vi "Report Data Update the Caller.vi"(8 "error in (no error)":errorcluster, 10 "Report Data":T1={"Schema"="", "Test Socket"="", "Start Test Cycle"="", "Stop Test Cycle"="", "Test Mode"="", "Frame Type"="fe_frame_log"}, 11 "Post Analysis in":refnum<class "Post Analysis.lvclass">) -> (0 "error out":errorcluster, 3 "Post Analysis out":refnum<class "Post Analysis.lvclass">)   [LabVIEW 2023, in "Data Analysis.lvlib" / "Post Analysis.lvlib" / "Post Analysis.lvclass"]
uses:
  Post Analysis.lvclass
  Control/Report.ctl
  Post Analysis.lvclass/Post Analysis.ctl
  Test Info/Test Info Messages/Report Data Update the Self Msg/Report Data Update the Self Msg.lvclass/Report Data Update the Self Msg.ctl
  <vilib>/ActorFramework/Message Enqueuer/Message Enqueuer.lvclass/Message Enqueuer.ctl
  Error Log/Error Log Messages/Result Data Update the Self Msg/Result Data Update the Self Msg.lvclass/Result Data Update the Self Msg.ctl
  FE FF Frame/FE FF Frame Messages/Result Data Update the Self Msg/Result Data Update the Self Msg.lvclass/Result Data Update the Self Msg.ctl
  Signal Analysis/Signal Analysis Messages/Result Data Update the Self Msg/Result Data Update the Self Msg.lvclass/Result Data Update the Self Msg.ctl
  Import Export/Import Export Messages/Result Data Update the Self Msg/Result Data Update the Self Msg.lvclass/Result Data Update the Self Msg.ctl
  Result Info/Result Info Messages/Result Data Update the Self Msg/Result Data Update the Self Msg.lvclass/Result Data Update the Self Msg.ctl
  <vilib>/ActorFramework/Message Enqueuer/Enqueue.vi
  Test Info/Test Info Messages/Report Data Update the Self Msg/Report Data Update the Self Msg.lvclass
  C:/Program Files/National Instruments/LabVIEW 2023/vi.lib/ActorFramework/Message/Message.lvclass
  Error Log/Error Log Messages/Result Data Update the Self Msg/Result Data Update the Self Msg.lvclass
  FE FF Frame/FE FF Frame Messages/Result Data Update the Self Msg/Result Data Update the Self Msg.lvclass
  Signal Analysis/Signal Analysis Messages/Result Data Update the Self Msg/Result Data Update the Self Msg.lvclass
  Signal Analysis/Signal Analysis Messages/Signal Name Update Msg/Signal Name Update Msg.lvclass
  Import Export/Import Export Messages/Result Data Update the Self Msg/Result Data Update the Self Msg.lvclass
  Result Info/Result Info Messages/Result Data Update the Self Msg/Result Data Update the Self Msg.lvclass
  <vilib>/ActorFramework/Message Priority Queue/Priority Enqueue.vi
  Data Analysis.lvlib
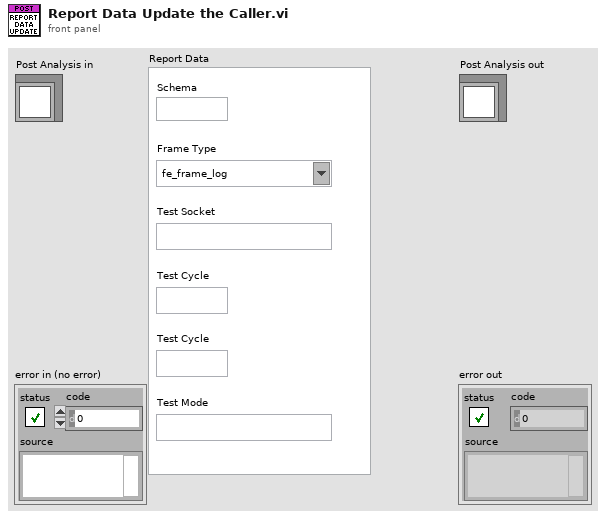
[diagram p1: front panel]
types:
  T1 = typedef "Data Analysis.lvlib/Report.ctl" = cluster{"Schema":string, "Test Socket":string, "Start Test Cycle":string, "Stop Test Cycle":string, "Test Mode":string, "Frame Type":string}
  T2 = enum32{"Test Info", "Error Log", "FE/FF Frame", "Signal Analysis", "Export", "Database", "Info"}
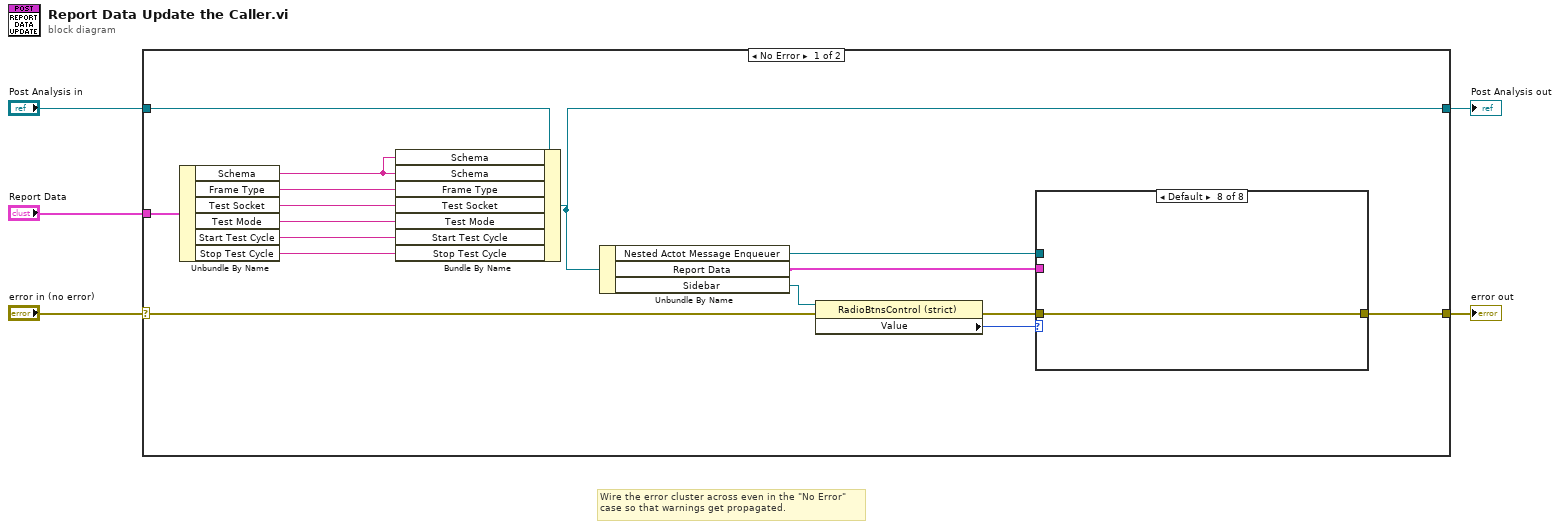
[diagram p0: block diagram]
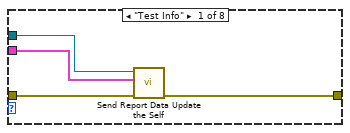
[diagram p2: hidden frame]
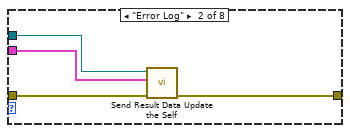
[diagram p3: hidden frame]
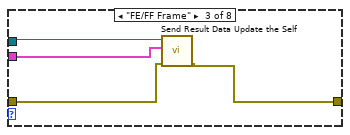
[diagram p4: hidden frame]
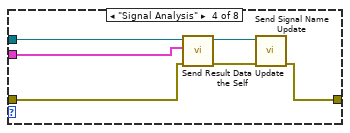
[diagram p5: hidden frame]
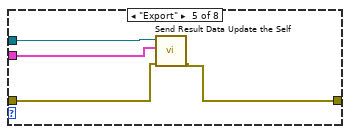
[diagram p6: hidden frame]
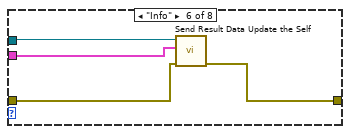
[diagram p7: hidden frame]
diagram:
  # "Wire the error cluster across even in the \"No Error\"\ncase so that warnings get propagated."
  n1 = case shown="No Error" "error in (no error)" {
    selector: "error in (no error)" -> [w8 w51]
    tunnel: [w11 w51] -> w4
    tunnel: [w14 w50] -> w2
    tunnel: "Post Analysis in" -> [w21 w50]
    tunnel: "Report Data" -> [w20 _]
    frame No Error {
      n2 = Unbundle By Name(w20) -> ("Schema"=w6:string, "Frame Type"=w19:string, "Test Socket"=w18:string, "Test Mode"=w17:string, "Start Test Cycle"=w16:string, "Stop Test Cycle"=w15:string)
      n3 = Bundle By Name(cluster=w21, "Schema"=w6, "Schema"=w6, "Frame Type"=w19, "Test Socket"=w18, "Test Mode"=w17, "Start Test Cycle"=w16, "Stop Test Cycle"=w15) -> (w14:refnum<class "Post Analysis.lvclass">)
      n4 = Unbundle By Name(w14) -> ("Nested Actot Message Enqueuer"=w13:refnum<class "Message Enqueuer.lvclass">, "Report Data"=w12:T1, "Sidebar"=w10:refnum<vi>)
      n5 = property class="RadioBtnsControl (strict)"(reference=w10, error in=w8) -> (error out=w7:errorcluster, "Value"=w9:T2)  [unwired: 1 out]
      n6 = case shown="Default" w9 {
        tunnel: w13 -> [w25 w29 w33 w39 w43 w47 _ _]
        tunnel: w12 -> [w24 w28 w32 w38 w42 w46 _ _]
        tunnel: w7 -> [w23 w27 w31 w37 w41 w45 w48 w49]
        tunnel: [w22 w26 w30 w34 w40 w44 w48 w49] -> w11
        frame "Test Info" {
          n7 = call "Send Report Data Update the Self.vi"("error in (no error)"=w23, "Report Data"=w24, "Message Enqueuer"=w25) -> ("error out"=w22:errorcluster)  [unwired: 7 in, 1 out]
        }
        frame "Error Log" {
          n8 = call "Send Result Data Update the Self.vi"("error in (no error)"=w27, "Report Data"=w28, "Message Enqueuer"=w29) -> ("error out"=w26:errorcluster)  [unwired: 7 in, 1 out]
        }
        frame "FE/FF Frame" {
          n9 = call "Send Result Data Update the Self.vi"("error in (no error)"=w31, "Report Data"=w32, "Message Enqueuer"=w33) -> ("error out"=w30:errorcluster)  [unwired: 7 in, 1 out]
        }
        frame "Signal Analysis" {
          n10 = call "Send Result Data Update the Self.vi"("error in (no error)"=w37, "Report Data"=w38, "Message Enqueuer"=w39) -> ("error out"=w35:errorcluster, "Message Enqueuer out"=w36:refnum<class "Message Enqueuer.lvclass">)  [unwired: 7 in]
          n11 = call "Send Signal Name Update.vi"("error in (no error)"=w35, "Message Enqueuer"=w36) -> ("error out"=w34:errorcluster)  [unwired: 8 in, 1 out]
        }
        frame "Export" {
          n12 = call "Send Result Data Update the Self.vi"("error in (no error)"=w41, "Report Data"=w42, "Message Enqueuer"=w43) -> ("error out"=w40:errorcluster)  [unwired: 7 in, 1 out]
        }
        frame "Info" {
          n13 = call "Send Result Data Update the Self.vi"("error in (no error)"=w45, "Report Data"=w46, "Message Enqueuer"=w47) -> ("error out"=w44:errorcluster)  [unwired: 7 in, 1 out]
        }
        frame "Database" {
        }
        frame Default {
        }
      }
    }
    frame Error {
    }
  }
  "error out" <- w4
  "Post Analysis out" <- w2
